vi "tsc_Search Ring.vi"(2 "Values":string[](array[string]), 3 "Search Item":string) -> (0 "Index":u16)   [LabVIEW 2021]
doc: "Look through the ring strings and find the match. If it isn't found, set to zero.\n\n<b>Code Developed By:</b>\nTechnology Service Corporation\n1983 S Liberty Drive\nBloomington, IN 47403\nPhone: 812 558-7100\nwww.tsc.com/atcs\n\nDeveloper:\nDaniel Coons"
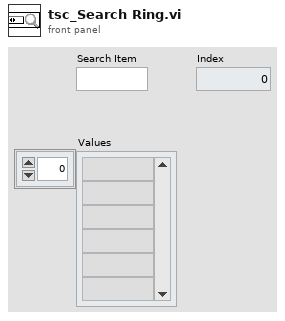
[diagram p1: front panel]
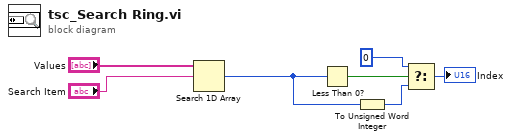
[diagram p0: block diagram]
diagram:
  n1 = Search 1D Array(1D array="Values", element="Search Item") -> (index of element=w2:i32)  [unwired: 1 in]
  n2 = Less Than 0?(x=w2) -> (x < 0?=w4:bool)
  n3 = To Unsigned Word Integer(number=w2) -> (unsigned 16bit integer=w1:u16)
  n4 = Select(t=u16 0, s=w4, f=w1) -> (s? t:f=→"Index":u16)
